vi "Loop_SM.vi"() -> ()   [LabVIEW 2017, in "MechamunDrive.lvlib"]
uses:
  MechamunDrive.lvlib
  Cluster_Auto Shut Off Ranges.ctl
  TypeDefs/Cluster_PID Constants Standard.ctl
  ENUM_State.ctl
  Enum_SM Cmd Select.ctl
  ENUM_Action.ctl
  Enum Tab_Select PID Mode.ctl
  Cluster_SM to HW Data.ctl
  Enum_HW Cmd Select.ctl
  Cluster_CMD to SM Data.ctl
  Cluster_HW Status.ctl
  TypeDefs/Cluster_SRX Status With Encoder.ctl
  VisionSystem/Cluster_Vision Status.ctl
  VisionSystem/Enum_ Field Targets.ctl
  Cluster_SM Status.ctl
  <vilib>/Rock Robotics/WPI/ThirdParty/Sensors/navX/_TypeDefs/FRIC_navX_DeviceNumbersTypeDef.ctl
  Global_CMD to SM Data.vi
  Sonar/Global_HW_Data Out.vi
  Global_HW_Status Out.vi
  VisionSystem/Global_Vision Status.vi
  _SHARE ALL/Global Share All/Global_STOP.vi
  <vilib>/addons/control/pid/pid.llb/PID (DBL).vi
  Global_SM Out Data.vi
  <vilib>/addons/control/pid/NI_PID_pid.lvlib
  Sonar/Sonar.lvlib
  VisionSystem/VisionSystem.lvlib
panel:
  out "Drive_HW_Status":T1
  out "SM Cmd":T3
  out "HW Cmd Out":T5
  in  "PID Select":T7
  in  "PID Track Rotation":T8={"proportional gain (Kc)"=0.005, "integral time (Ti, min)"=0.0, "derivative time (Td, min)"=0.0028} {"derivative time (Td, min)" format="%.5f"; "integral time (Ti, min)" format="%.5f"; "proportional gain (Kc)" format="%.5f"}
  in  "PID Lock Angle Rotation":T8={"proportional gain (Kc)"=0.012, "integral time (Ti, min)"=0.0, "derivative time (Td, min)"=0.002} {"derivative time (Td, min)" format="%.5f"; "integral time (Ti, min)" format="%.5f"; "proportional gain (Kc)" format="%.5f"}
  in  "PID Track Lateral":T8={"proportional gain (Kc)"=0.05, "integral time (Ti, min)"=0.0, "derivative time (Td, min)"=0.0} {"derivative time (Td, min)" format="%.5f"; "integral time (Ti, min)" format="%.5f"; "proportional gain (Kc)" format="%.5f"}
  in  "PID Track Vision Lat":T8={"proportional gain (Kc)"=0.03, "integral time (Ti, min)"=0.0, "derivative time (Td, min)"=0.0} {"derivative time (Td, min)" format="%.5f"; "integral time (Ti, min)" format="%.5f"; "proportional gain (Kc)" format="%.5f"}
  in  "lateral f":dbl=0.1 format="%#_13g"
  in  "PID Track Vision Rot":T8={"proportional gain (Kc)"=0.0015, "integral time (Ti, min)"=0.0, "derivative time (Td, min)"=0.0} {"derivative time (Td, min)" format="%.5f"; "integral time (Ti, min)" format="%.5f"; "proportional gain (Kc)" format="%.5f"}
  in  "Vision Track target":dbl=8.0 format="%#_13g"
  in  "PID Track Front":T8={"proportional gain (Kc)"=0.005, "integral time (Ti, min)"=0.0, "derivative time (Td, min)"=0.0} {"derivative time (Td, min)" format="%.5f"; "integral time (Ti, min)" format="%.5f"; "proportional gain (Kc)" format="%.5f"}
  out "Action":T9
  out "CMDMODE":T4
  out "Complete":bool
  out "PID Output":dbl
  out "PID Reading":dbl
  out "PID Target":dbl
  out "Cycle Time":dbl
  out "State":T10
  out "Output":dbl(graph)
  out "Process Chart":cluster{"PID Target":dbl, "PID Reading":dbl}(graph)
  in  "Auto Shut Off Ranges":T11={"Track Front Back"=1.0, "Track Rotation"=1.0, "Track Lateral"=1.0, "Track Vision"=2.0}
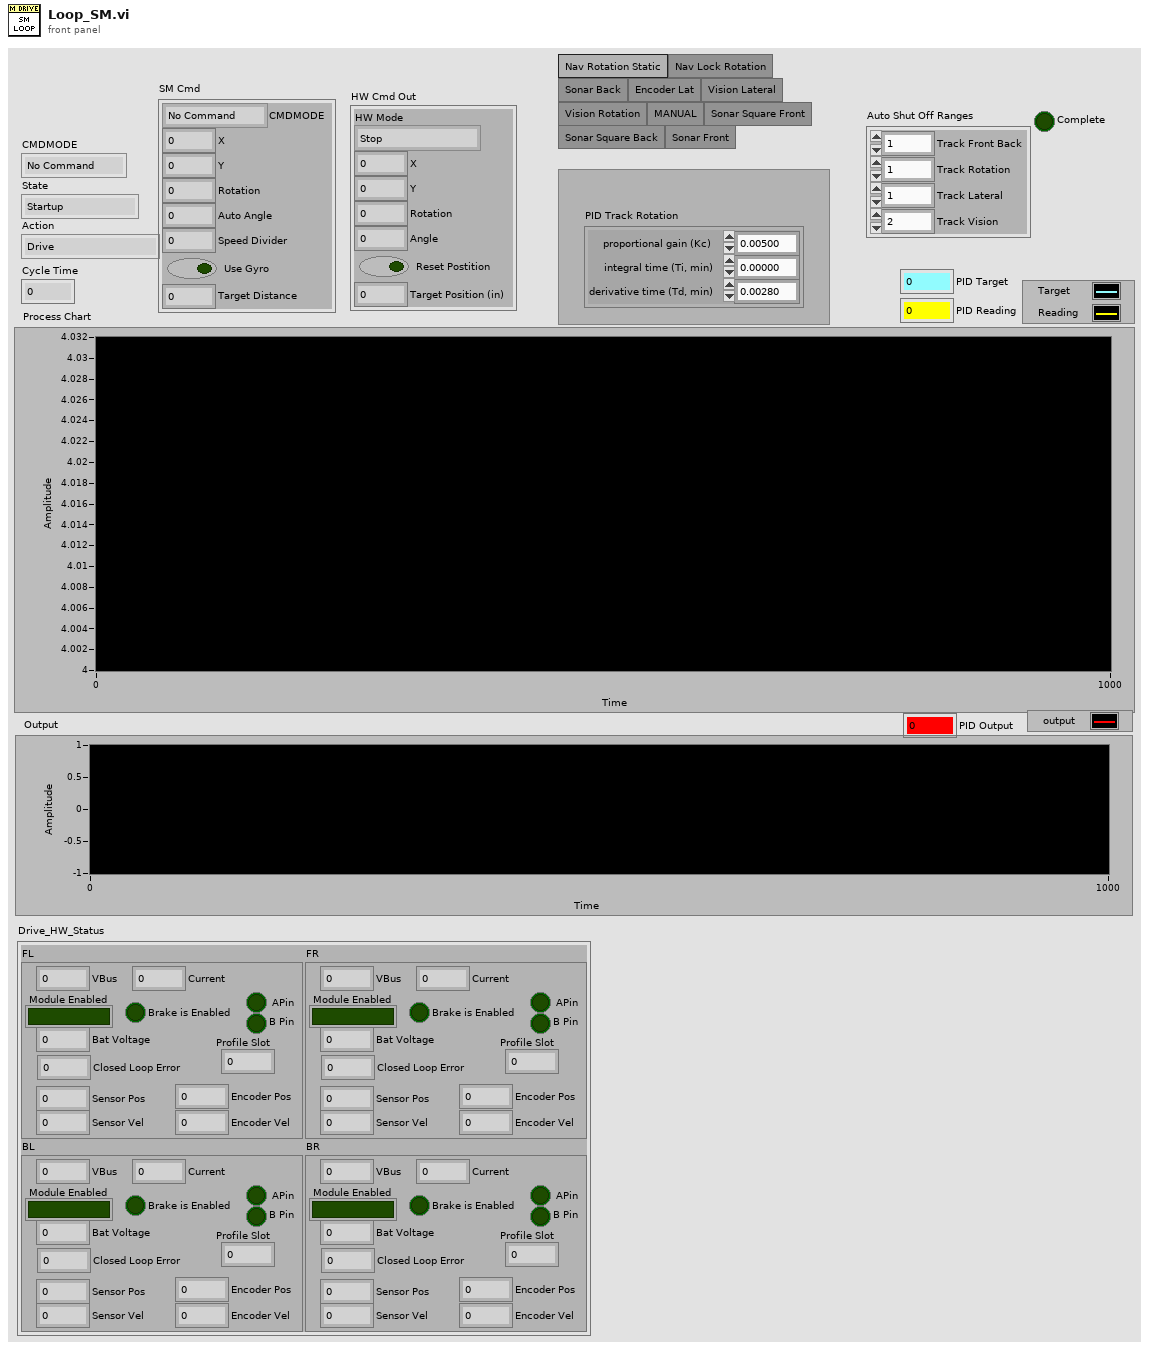
[diagram p1: front panel]
types:
  T1 = typedef "MechamunDrive.lvlib/Cluster_HW Status.ctl" = cluster{"BL":T2, "BR":T2, "FL":T2, "FR":T2}
  T2 = typedef "Cluster_SRX Status With Encoder.ctl" = cluster{"VBus ":dbl, "Module Enabled":bool, "Closed Loop Error":dbl, "Sensor Pos":dbl, "Sensor Vel":dbl, "Current":dbl, "Brake is Enabled":bool, "Encoder Pos":dbl, "Encoder Vel":dbl, " APin":bool, "B Pin":bool, "Bat Voltage":dbl, "Profile Slot":dbl}
  T3 = typedef "MechamunDrive.lvlib/Cluster_CMD to SM Data.ctl" = cluster{"CMDMODE":T4, "X":dbl, "Y":dbl, "Rotation":dbl, "Auto Angle":dbl, "Speed Divider":dbl, "Use Gyro":bool, "Target Distance":dbl}
  T4 = typedef "MechamunDrive.lvlib/Enum_SM Cmd Select.ctl" = enum16{"No Command", "Halt", "Manual Keep Rotation", "Manual", "Track Front", "Track Rotation", "Track Lateral", "Track Vision Lat", "Track Vision Rot", "Strafe Right", "Strafe Left"}
  T5 = typedef "MechamunDrive.lvlib/Cluster_SM to HW Data.ctl" = cluster{"HW Mode":T6, "X":dbl, "Y":dbl, "Rotation":dbl, "Angle":dbl, "Reset Postition":bool, "Target Position (in)":dbl}
  T6 = typedef "MechamunDrive.lvlib/Enum_HW Cmd Select.ctl" = enum16{"Stop", "Vbus", "Positon Lateral", "Postition  FrontBack"}
  T7 = typedef "MechamunDrive.lvlib/Enum Tab_Select PID Mode.ctl" = enum32{"Nav Rotation Static", "Nav Lock Rotation", "Sonar Back", "Encoder Lat", "Vision Lateral", "Vision Rotation", "MANUAL", "Sonar Square Front", "Sonar Square Back", "Sonar Front"}
  T8 = typedef "Cluster_PID Constants Standard.ctl" = cluster{"proportional gain (Kc)":dbl, "integral time (Ti, min)":dbl, "derivative time (Td, min)":dbl}
  T9 = typedef "MechamunDrive.lvlib/ENUM_Action.ctl" = enum16{"Drive", "Strafe Left", "Strafe Right", "No Action", "Manuel Keep Rotation", "Reset Time", "Stop Move", "Track Front Distance", "Set Lock Angle", "Reset Gyro", "Track Rotation", "Track Lateral Encoders", "NavX Pos Reset", "Track Vision Lat", "Track Vision Rot", "Reset Position"}
  T10 = typedef "MechamunDrive.lvlib/ENUM_State.ctl" = enum16{"Startup", "Idle", "Manual", "Rotation Tracking", "Distance Tracking", "Shutdown", "Lateral Tracking", "Vision Tracking Lat", "Vision Tracking Rot", "Strafing", "Manual Keep Rotation", "Halt"}
  T11 = typedef "MechamunDrive.lvlib/Cluster_Auto Shut Off Ranges.ctl" = cluster{"Track Front Back":dbl, "Track Rotation":dbl, "Track Lateral":dbl, "Track Vision":dbl}
  T12 = typedef "MechamunDrive.lvlib/Cluster_SM Status.ctl" = cluster{"Drive Cmd":T4, "Complete":bool}
  T13 = typedef "VisionSystem.lvlib/Cluster_Vision Status.ctl" = cluster{"Target Found":bool, "Target":T14, "Pixels to Center":dbl, "Vision Distance Center (in)":dbl, "Angle Distance Center (in)":dbl}
  T14 = typedef "VisionSystem.lvlib/Enum_ Field Targets.ctl" = enum16{"Boiler (USB 0)", "Rope (USB 1)"}
  T15 = cluster{"Velocity X":dbl, "Velocity Y":dbl, "Velocity Z":dbl, "Displacement X":dbl, "Displacement Y":dbl, "Displacement Z":dbl}
  T16 = cluster{"Actions":T9[], "State":T10, "Current Time":timestamp, "Start Time":timestamp, "Loop Time (ms)":u32, "CMD Drive":T3, "Set Angle Out":dbl, "Sonar Distance":dbl, "Lock Angle":dbl, "previous State":T10, "Position Data":cluster{"Velocity X":dbl, "Velocity Y":dbl, "Velocity Z":dbl, "Displacement X":dbl, "Displacement Y":dbl, "Displacement Z":dbl}, "Vision Data":T13, "Shut Off Ranges":T11, "Status OUT":T12, "PID Target":dbl, "PID Reading":dbl, "PID Output":dbl, "DriveHWCmd OUT":T5, "Gyro Angle":dbl, "Drive HW Status":T1, "Lateral Distance":dbl, "PID Select":T7}
  T17 = typedef "FRIC_navX_DeviceNumbersTypeDef.ctl" = enum16{"Dev0", "Dev1", "Dev2", "Dev3"}
  T18 = cluster{"Yaw":dbl, "Roll":dbl, "Pitch":dbl, "Heading":dbl, "Fused Heading":dbl}
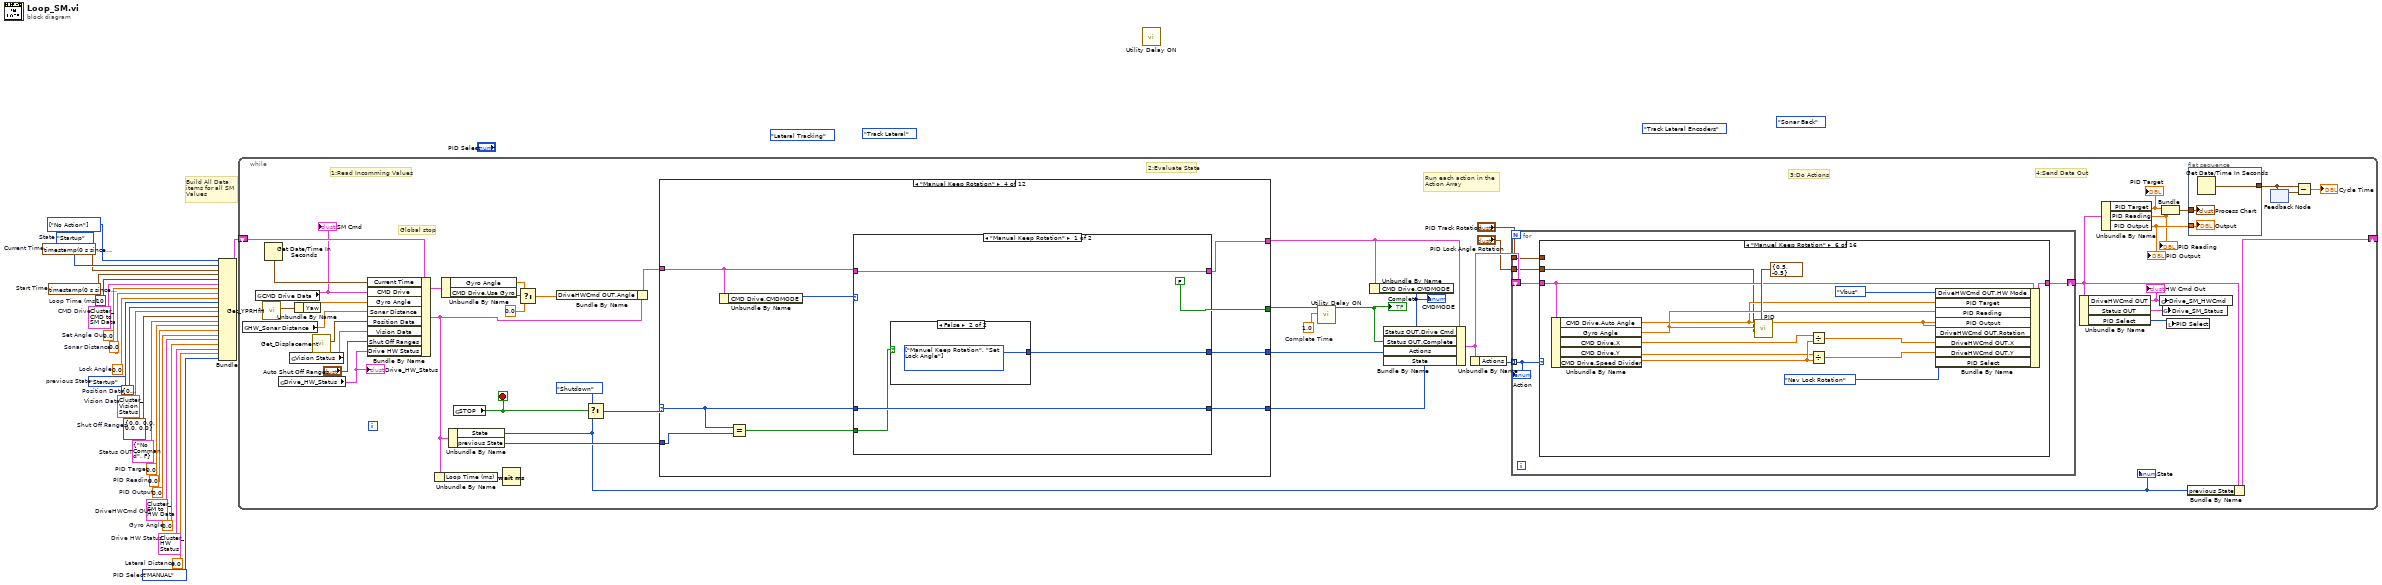
[diagram p0: block diagram]
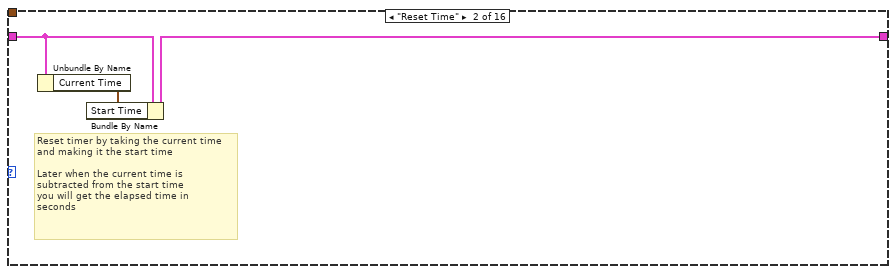
[diagram p3: hidden frame]
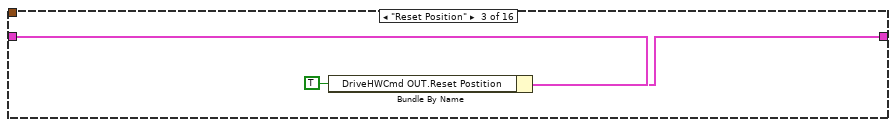
[diagram p4: hidden frame]
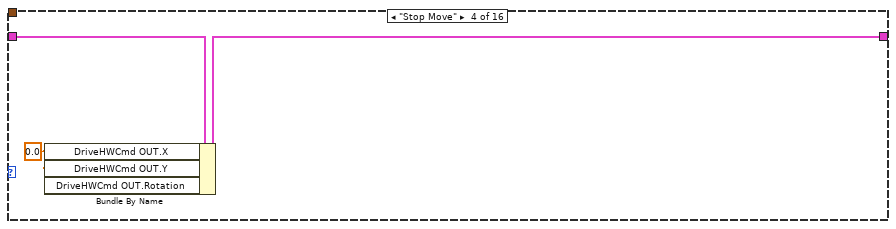
[diagram p5: hidden frame]
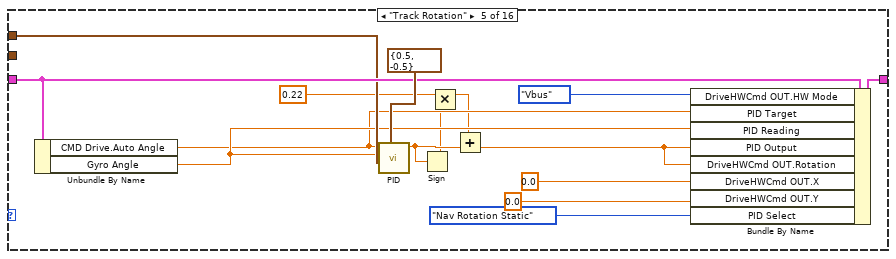
[diagram p6: hidden frame]
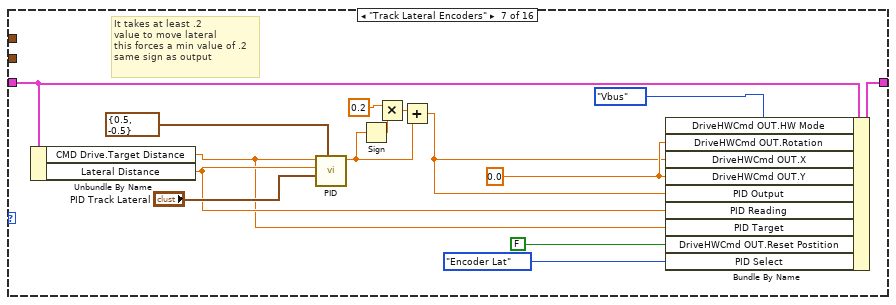
[diagram p7: hidden frame]
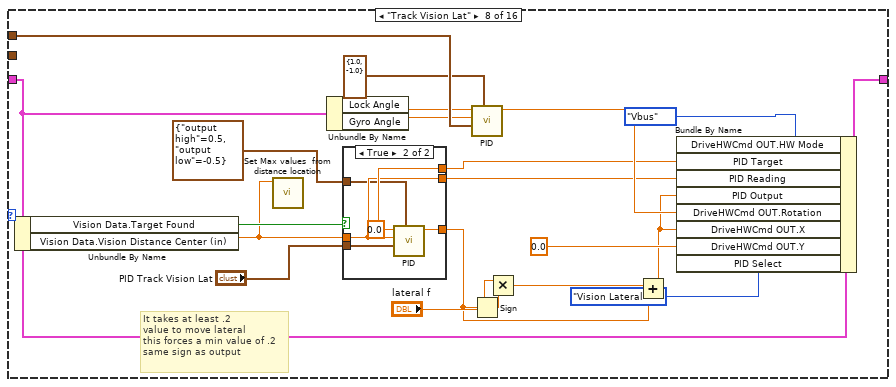
[diagram p8: hidden frame]
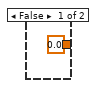
[diagram p9: hidden frame]
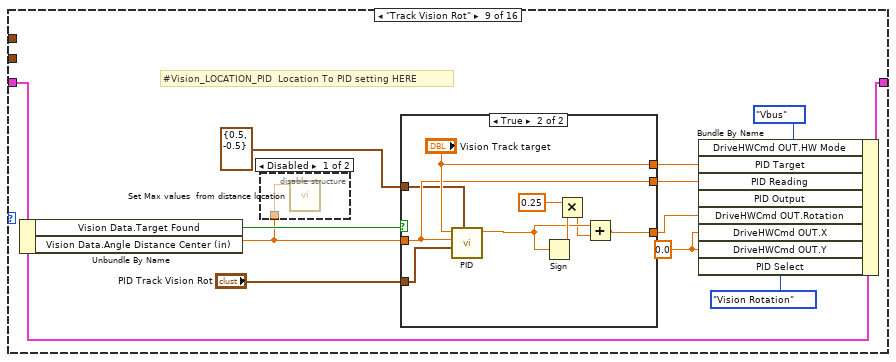
[diagram p10: hidden frame]
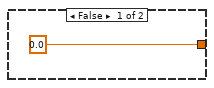
[diagram p12: hidden frame]
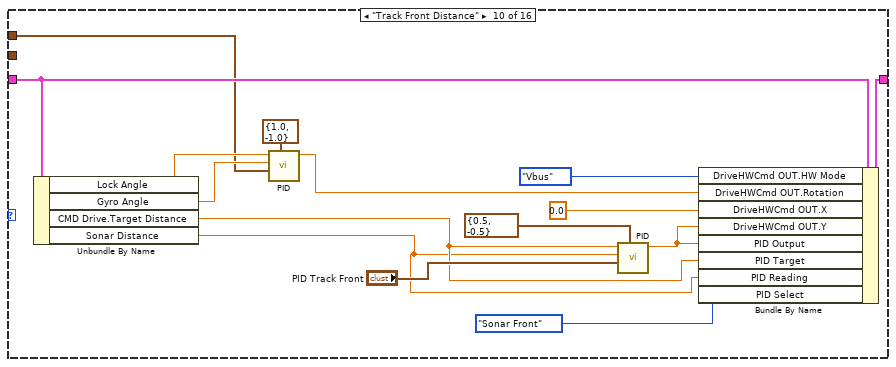
[diagram p13: hidden frame]
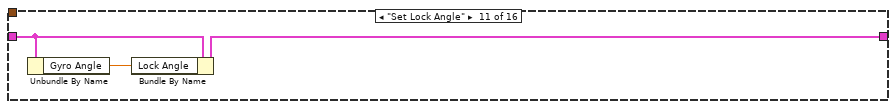
[diagram p14: hidden frame]
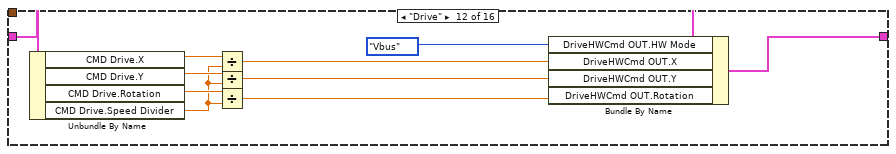
[diagram p15: hidden frame]
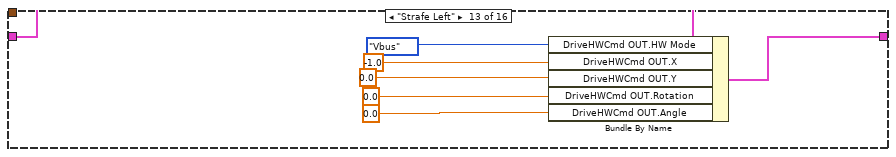
[diagram p16: hidden frame]
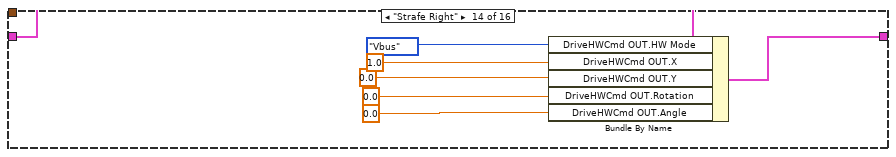
[diagram p17: hidden frame]
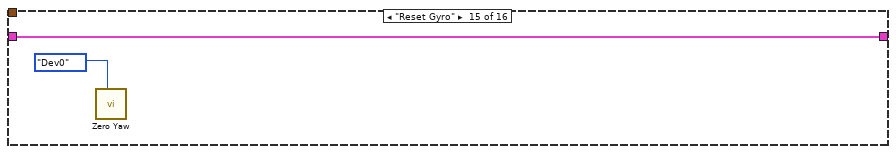
[diagram p18: hidden frame]
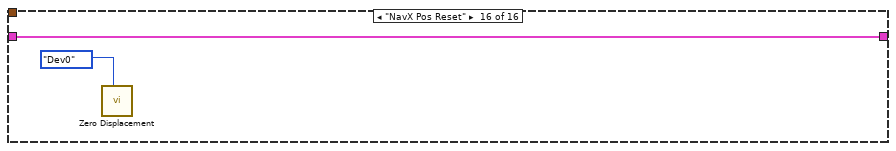
[diagram p19: hidden frame]
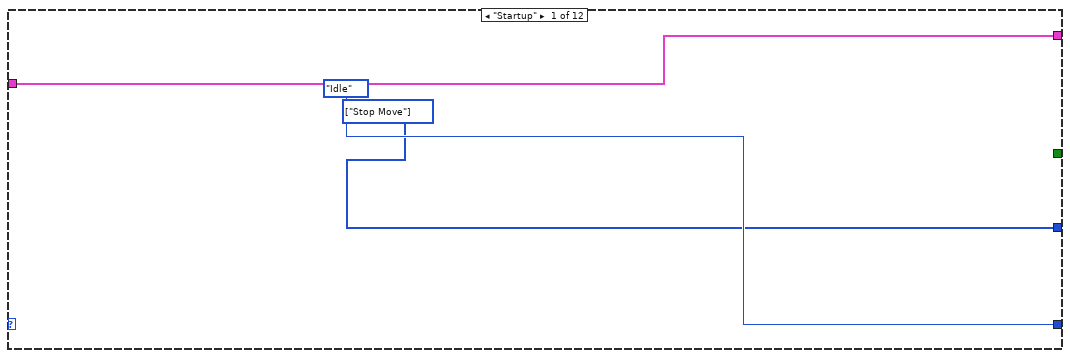
[diagram p20: hidden frame]
diagram:
  (unwired) Enum_SM_Cmd_Select."Track Lateral" ("CMD Drive.CMDMODE")
  (unwired) Enum_Tab_Select_PID_Mode."Sonar Back" ("PID Select")
  (unwired) ENUM_Action."Track Lateral Encoders" ("Action")
  (unwired) ENUM_State."Lateral Tracking" ("State")
  w1 = 0.0  # Sonar Distance
  w2 = Enum_Tab_Select_PID_Mode."MANUAL"  # PID Select
  w3 = 0.0  # Lateral Distance
  w4 = T1 {"BL"={"VBus "=0.0, "Module Enabled"=FALSE, "Closed Loop Error"=0.0, "Sensor Pos"=0.0, "Sensor Vel"=0.0, "Current"=0.0, "Brake is Enabled"=FALSE, "Encoder Pos"=0.0, "Encoder Vel"=0.0, " APin"=FALSE, "B Pin"=FALSE, "Bat Voltage"=0.0, "Profile Slot"=0.0}, "BR"={"VBus "=0.0, "Module Enabled"=FALSE, "Closed Loop Error"=0.0, "Sensor Pos"=0.0, "Sensor Vel"=0.0, "Current"=0.0, "Brake is Enabled"=FALSE, "Encoder Pos"=0.0, "Encoder Vel"=0.0, " APin"=FALSE, "B Pin"=FALSE, "Bat Voltage"=0.0, "Profile Slot"=0.0}, "FL"={"VBus "=0.0, "Module Enabled"=FALSE, "Closed Loop Error"=0.0, "Sensor Pos"=0.0, "Sensor Vel"=0.0, "Current"=0.0, "Brake is Enabled"=FALSE, "Encoder Pos"=0.0, "Encoder Vel"=0.0, " APin"=FALSE, "B Pin"=FALSE, "Bat Voltage"=0.0, "Profile Slot"=0.0}, "FR"={"VBus "=0.0, "Module Enabled"=FALSE, "Closed Loop Error"=0.0, "Sensor Pos"=0.0, "Sensor Vel"=0.0, "Current"=0.0, "Brake is Enabled"=FALSE, "Encoder Pos"=0.0, "Encoder Vel"=0.0, " APin"=FALSE, "B Pin"=FALSE, "Bat Voltage"=0.0, "Profile Slot"=0.0}}  # Drive HW Status
  w5 = 0.0  # Gyro Angle
  w6 = T5 {"HW Mode"=enum."Postition  FrontBack", "X"=0.0, "Y"=0.0, "Rotation"=0.0, "Angle"=0.0, "Reset Postition"=FALSE, "Target Position (in)"=0.0}  # DriveHWCmd OUT
  w7 = 0.0  # PID Output
  w8 = 0.0  # PID Reading
  w9 = 0.0  # PID Target
  w10 = T12 {"Drive Cmd"=enum."No Command", "Complete"=FALSE}  # Status OUT
  w11 = T11 {"Track Front Back"=0.0, "Track Rotation"=0.0, "Track Lateral"=0.0, "Track Vision"=0.0}  # Shut Off Ranges
  w12 = T13 {"Target Found"=FALSE, "Target"=enum."Boiler (USB 0)", "Pixels to Center"=0.0, "Vision Distance Center (in)"=0.0, "Angle Distance Center (in)"=0.0}  # Vision Data
  w13 = T15 {"Velocity X"=0.0, "Velocity Y"=0.0, "Velocity Z"=0.0, "Displacement X"=0.0, "Displacement Y"=0.0, "Displacement Z"=0.0}  # Position Data
  w14 = ENUM_State."Startup"  # previous State
  w15 = 0.0  # Lock Angle
  w16 = 0.0  # Set Angle Out
  w17 = T3 {"CMDMODE"=enum."No Command", "X"=0.0, "Y"=0.0, "Rotation"=0.0, "Auto Angle"=0.0, "Speed Divider"=0.0, "Use Gyro"=FALSE, "Target Distance"=0.0}  # CMD Drive
  w18 = u32 10  # Loop Time (ms)
  w19 = T9[] [enum."No Action"] items=["Drive", "Strafe Left", "Strafe Right", "No Action", "Manuel Keep Rotation", "Reset Time", "Stop Move", "Track Front Distance", "Set Lock Angle", "Reset Gyro", "Track Rotation", "Track Lateral Encoders", "NavX Pos Reset", "Track Vision Lat", "Track Vision Rot", "Reset Position"] ("Actions")
  w20 = timestamp(0 s since 1904-01-01)  # Start Time
  w21 = timestamp(0 s since 1904-01-01)  # Current Time
  w22 = ENUM_State."Startup"  # State
  # "Build All Data items for all SM Values"
  n1 = Bundle("Actions"=w19, "State"=w22, "Current Time"=w21, "Start Time"=w20, "Loop Time (ms)"=w18, "CMD Drive"=w17, "Set Angle Out"=w16, "Sonar Distance"=w1, "Lock Angle"=w15, "previous State"=w14, "Position Data"=w13, "Vision Data"=w12, "Shut Off Ranges"=w11, "Status OUT"=w10, "PID Target"=w9, "PID Reading"=w8, "PID Output"=w7, "DriveHWCmd OUT"=w6, "Gyro Angle"=w5, "Drive HW Status"=w4, "Lateral Distance"=w3, "PID Select"=w2) -> (w23:T16)  [unwired: 1 in]
  n2 = while {
    shift-right: [w48] -> _
    shift-left: w23 -> [w67]
    stop <- w64 stop-if-true
    w24 = 1.0  # Complete Time
    # "Run each action in the Action Array"
    # "1:Read Incomming Values"
    # "2:Evaluate State"
    # "3:Do Actions"
    # "4:Send Data Out"
    # "Global stop"
    n3 = global read "Global_HW_Data Out.vi" "HW_Sonar Distance"() -> (w27:dbl)
    n4 = global read "Global_CMD to SM Data.vi" "CMD Drive Data"() -> (w60:T3)
    "SM Cmd" <- w60
    n5 = call <vilib>:"Get_YPRHfH.vi"() -> ("YRPHfH"=w59:T18)  [unwired: 11 in]
    n6 = Get Date/Time In Seconds() -> (seconds since 1Jan1904=w66:timestamp)
    n7 = global read "Global_HW_Status Out.vi" "Drive_HW_Status"() -> (w29:T1)
    "Drive_HW_Status" <- w29
    n8 = global read "Global_Vision Status.vi" "Vision Status"() -> (w46:T13)
    n9 = Unbundle By Name(w59) -> ("Yaw"=w57:dbl)
    n10 = call <vilib>:"Get_Displacement.vi"() -> ("Displacement"=w47:T15)  [unwired: 11 in]
    n11 = Bundle By Name(cluster=w67, "Current Time"=w66, "CMD Drive"=w60, "Gyro Angle"=w57, "Sonar Distance"=w27, "Position Data"=w47, "Vision Data"=w46, "Shut Off Ranges"="Auto Shut Off Ranges", "Drive HW Status"=w29) -> (w52:T16)
    n12 = Unbundle By Name(w52) -> ("Loop Time (ms)"=w61:u32)
    n13 = Unbundle By Name(w52) -> ("Gyro Angle"=w54:dbl, "CMD Drive.Use Gyro"=w55:bool)
    n14 = Unbundle By Name(w52) -> ("State"=w45:T10, "previous State"=w49:T10)
    "State" <- w45
    n15 = global read "Global_STOP.vi" "STOP"() -> (w64:bool)
    n16 = Wait (ms)(milliseconds to wait=w61) -> ()  [unwired: 1 out]
    n17 = Select(t=w54, s=w55, f=0.0) -> (s? t:f=w50:dbl)
    n18 = Bundle By Name(cluster=w52, "DriveHWCmd OUT.Angle"=w50) -> (w51:T16)
    n19 = Select(t=ENUM_State."Shutdown" ("State"), s=w64, f=w45) -> (s? t:f=w62:T10)
    n20 = case shown="\"Manual Keep Rotation\"" w62 {
      selector: w62 -> [_ _ w260 w271 w287 w309 w352 w386 w412 _ _ _]
      tunnel: w51 -> [w229 w232 w256 w272 w292 w314 w357 w391 w416 w434 w438 w446]
      tunnel: [w229 w231 w257 w273 w291 w315 w358 w392 w415 w434 w438 w446] -> w42
      tunnel: [ENUM_State."Idle" ("State") w230 w259 w275 w290 w313 w356 w390 w411 ENUM_State."Shutdown" ("State") w435 w445] -> w40
      tunnel: [w227 _ w258 w274 w289 w312 w355 w389 w413 w432 w436 w448] -> w58
      tunnel: w49 -> [_ _ _ w270 _ w310 w353 w387 _ _ _ _]
      tunnel: [_ _ FALSE FALSE w288 w311 w354 w388 w414 _ _ _] -> w25
      frame "Startup" {
        w227 = T9[] [enum."Stop Move"] items=["Drive", "Strafe Left", "Strafe Right", "No Action", "Manuel Keep Rotation", "Reset Time", "Stop Move", "Track Front Distance", "Set Lock Angle", "Reset Gyro", "Track Rotation", "Track Lateral Encoders", "NavX Pos Reset", "Track Vision Lat", "Track Vision Rot", "Reset Position"] ("Actions")
      }
      frame "Idle" {
        # "For each call of the state\nDecide next State and set\nActions"
        # "What will the next state be"
        n21 = Unbundle By Name(w232) -> ("CMD Drive.CMDMODE"=w233:T4)
        n22 = case shown="\"Halt\"" w233 {
          tunnel: w232 -> [w234 w236 w239 w240 w243 w245 w247 w249 w250 w253 w255]
          tunnel: [w234 w236 w239 w240 w243 w245 w247 w249 w250 w253 w255] -> w231
          tunnel: [ENUM_State."Idle" ("State") ENUM_State."Rotation Tracking" ("State") ENUM_State."Manual Keep Rotation" ("State") ENUM_State."Distance Tracking" ("State") ENUM_State."Lateral Tracking" ("State") ENUM_State."Manual" ("State") ENUM_State."Vision Tracking Lat" ("State") ENUM_State."Vision Tracking Rot" ("State") ENUM_State."Strafing" ("State") ENUM_State."Strafing" ("State") ENUM_State."Halt" ("State")] -> w230
          frame "No Command" {
          }
          frame "Track Rotation" {
          }
          frame "Manual Keep Rotation" {
          }
          frame "Track Front" {
          }
          frame "Track Lateral" {
          }
          frame "Manual" {
          }
          frame "Track Vision Lat" {
          }
          frame "Track Vision Rot" {
          }
          frame "Strafe Right" {
          }
          frame "Strafe Left" {
          }
          frame "Halt" {
          }
        }
      }
      frame "Manual" {
        n23 = Unbundle By Name(w256) -> ("CMD Drive.CMDMODE"=w261:T4)
        n24 = case shown="\"Manual\"" w261 {
          tunnel: w256 -> [w264 w268]
          tunnel: [w264 w268] -> w257
          tunnel: [w263 ENUM_State."Idle" ("State")] -> w259
          tunnel: [w265 w266] -> w258
          tunnel: w260 -> [w263 _]
          frame "Manual" {
            w265 = T9[] [enum."Drive"] items=["Drive", "Strafe Left", "Strafe Right", "No Action", "Manuel Keep Rotation", "Reset Time", "Stop Move", "Track Front Distance", "Set Lock Angle", "Reset Gyro", "Track Rotation", "Track Lateral Encoders", "NavX Pos Reset", "Track Vision Lat", "Track Vision Rot", "Reset Position"] ("Actions")
          }
          frame Default {
            w266 = T9[] [enum."Stop Move"] items=["Drive", "Strafe Left", "Strafe Right", "No Action", "Manuel Keep Rotation", "Reset Time", "Stop Move", "Track Front Distance", "Set Lock Angle", "Reset Gyro", "Track Rotation", "Track Lateral Encoders", "NavX Pos Reset", "Track Vision Lat", "Track Vision Rot", "Reset Position"] ("Actions")
          }
        }
      }
      frame "Manual Keep Rotation" {
        n25 = Unbundle By Name(w272) -> ("CMD Drive.CMDMODE"=w276:T4)
        n26 = Equal?(x=w271, y=w270) -> (x = y?=w269:bool)
        n27 = case shown="\"Manual Keep Rotation\"" w276 {
          tunnel: w272 -> [w280 w286]
          tunnel: [w280 w286] -> w273
          tunnel: [w279 ENUM_State."Idle" ("State")] -> w275
          tunnel: [w281 w284] -> w274
          tunnel: w271 -> [w279 _]
          tunnel: w269 -> [w278 _]
          frame "Manual Keep Rotation" {
            n28 = case shown="False" w278 {
              tunnel: [w282 w283] -> w281
              frame True {
                w282 = T9[] [enum."Manuel Keep Rotation"] items=["Drive", "Strafe Left", "Strafe Right", "No Action", "Manuel Keep Rotation", "Reset Time", "Stop Move", "Track Front Distance", "Set Lock Angle", "Reset Gyro", "Track Rotation", "Track Lateral Encoders", "NavX Pos Reset", "Track Vision Lat", "Track Vision Rot", "Reset Position"] ("Actions")
              }
              frame False {
                w283 = T9[] [enum."Manuel Keep Rotation", enum."Set Lock Angle"] items=["Drive", "Strafe Left", "Strafe Right", "No Action", "Manuel Keep Rotation", "Reset Time", "Stop Move", "Track Front Distance", "Set Lock Angle", "Reset Gyro", "Track Rotation", "Track Lateral Encoders", "NavX Pos Reset", "Track Vision Lat", "Track Vision Rot", "Reset Position"] ("Actions")
              }
            }
          }
          frame Default {
            w284 = T9[] [enum."Stop Move"] items=["Drive", "Strafe Left", "Strafe Right", "No Action", "Manuel Keep Rotation", "Reset Time", "Stop Move", "Track Front Distance", "Set Lock Angle", "Reset Gyro", "Track Rotation", "Track Lateral Encoders", "NavX Pos Reset", "Track Vision Lat", "Track Vision Rot", "Reset Position"] ("Actions")
          }
        }
      }
      frame "Rotation Tracking" {
        n29 = Unbundle By Name(w292) -> ("CMD Drive.CMDMODE"=w293:T4)
        n30 = case shown="Default" w293 {
          tunnel: w292 -> [w295 w307]
          tunnel: [w295 w307] -> w291
          tunnel: [w297 ENUM_State."Idle" ("State")] -> w290
          tunnel: [w296 w305] -> w289
          tunnel: [w294 _] -> w288
          tunnel: w287 -> [w297 _]
          frame "Track Rotation" {
            n31 = Unbundle By Name(w295) -> ("CMD Drive.Auto Angle"=w301:dbl, "Gyro Angle"=w302:dbl, "Shut Off Ranges.Track Rotation"=w299:dbl)
            n32 = Subtract(x=w301, y=w302) -> (x-y=w300:dbl)
            n33 = Absolute Value(x=w300) -> (abs(x)=w298:dbl)
            n34 = Less Or Equal?(x=w298, y=w299) -> (x <= y?=w294:bool)
            n35 = case shown="True" w294 {
              tunnel: [w303 w304] -> w296
              frame False {
                w303 = T9[] [enum."Track Rotation"] items=["Drive", "Strafe Left", "Strafe Right", "No Action", "Manuel Keep Rotation", "Reset Time", "Stop Move", "Track Front Distance", "Set Lock Angle", "Reset Gyro", "Track Rotation", "Track Lateral Encoders", "NavX Pos Reset", "Track Vision Lat", "Track Vision Rot", "Reset Position"] ("Actions")
              }
              frame True {
                w304 = T9[] [enum."Stop Move"] items=["Drive", "Strafe Left", "Strafe Right", "No Action", "Manuel Keep Rotation", "Reset Time", "Stop Move", "Track Front Distance", "Set Lock Angle", "Reset Gyro", "Track Rotation", "Track Lateral Encoders", "NavX Pos Reset", "Track Vision Lat", "Track Vision Rot", "Reset Position"] ("Actions")
              }
            }
          }
          frame Default {
            w305 = T9[] [enum."Stop Move"] items=["Drive", "Strafe Left", "Strafe Right", "No Action", "Manuel Keep Rotation", "Reset Time", "Stop Move", "Track Front Distance", "Set Lock Angle", "Reset Gyro", "Track Rotation", "Track Lateral Encoders", "NavX Pos Reset", "Track Vision Lat", "Track Vision Rot", "Reset Position"] ("Actions")
          }
        }
      }
      frame "Lateral Tracking" {
        n36 = Unbundle By Name(w314) -> ("CMD Drive.CMDMODE"=w316:T4)
        n37 = Not Equal?(x=w309, y=w310) -> (x != y?=w308:bool)
        n38 = case shown="\"Track Lateral\"" w316 {
          tunnel: w314 -> [w319 w350]
          tunnel: [w318 w350] -> w315
          tunnel: [w321 ENUM_State."Idle" ("State")] -> w313
          tunnel: [w322 w348] -> w312
          tunnel: [w320 _] -> w311
          tunnel: w309 -> [w321 _]
          tunnel: w308 -> [w317 _]
          frame "Track Lateral" {
            n39 = case shown="False" w317 {
              tunnel: [w330 w347] -> w322
              tunnel: [w329 FALSE] -> w320
              tunnel: w319 -> [w325 w346]
              tunnel: [w327 w346] -> w318
              frame False {
                # "Previous \nSame"
                n40 = Unbundle By Name(w325) -> ("Drive HW Status"=w328:T1)
                n41 = call "Calculate Position.vi"("Drive HW Status"=w328) -> ("Reset"=w326:bool, "Distance"=w323:dbl)  [unwired: 8 in, 1 out]
                n42 = Bundle By Name(cluster=w325, "Lateral Distance"=w323) -> (w324:T16)
                n43 = case shown="False" w326 {
                  tunnel: [w339 w343] -> w330
                  tunnel: w324 -> [w332 w344]
                  tunnel: [w333 _] -> w329
                  tunnel: [w332 w344] -> w327
                  tunnel: w323 -> [w331 _]
                  frame False {
                    # "Encoders have value"
                    n44 = Unbundle By Name(w332) -> ("CMD Drive.Target Distance"=w338:dbl, "Shut Off Ranges.Track Lateral"=w336:dbl)
                    n45 = Subtract(x=w338, y=w331) -> (x-y=w337:dbl)
                    n46 = Absolute Value(x=w337) -> (abs(x)=w334:dbl)
                    n47 = Less Or Equal?(x=w334, y=w336) -> (x <= y?=w335:bool)
                    n48 = case shown="False" w335 {
                      tunnel: [w340 w342] -> w339
                      tunnel: [_ TRUE] -> w333
                      frame False {
                        w340 = T9[] [enum."Track Lateral Encoders"] items=["Drive", "Strafe Left", "Strafe Right", "No Action", "Manuel Keep Rotation", "Reset Time", "Stop Move", "Track Front Distance", "Set Lock Angle", "Reset Gyro", "Track Rotation", "Track Lateral Encoders", "NavX Pos Reset", "Track Vision Lat", "Track Vision Rot", "Reset Position"] ("Actions")
                      }
                      frame True {
                        w342 = T9[] [enum."Stop Move"] items=["Drive", "Strafe Left", "Strafe Right", "No Action", "Manuel Keep Rotation", "Reset Time", "Stop Move", "Track Front Distance", "Set Lock Angle", "Reset Gyro", "Track Rotation", "Track Lateral Encoders", "NavX Pos Reset", "Track Vision Lat", "Track Vision Rot", "Reset Position"] ("Actions")
                      }
                    }
                  }
                  frame True {
                    w343 = T9[] [enum."Drive", enum."Track Lateral Encoders"] items=["Drive", "Strafe Left", "Strafe Right", "No Action", "Manuel Keep Rotation", "Reset Time", "Stop Move", "Track Front Distance", "Set Lock Angle", "Reset Gyro", "Track Rotation", "Track Lateral Encoders", "NavX Pos Reset", "Track Vision Lat", "Track Vision Rot", "Reset Position"] ("Actions")
                    # "Encoder are Reset"
                  }
                }
              }
              frame True {
                w347 = T9[] [enum."Reset Position"] items=["Drive", "Strafe Left", "Strafe Right", "No Action", "Manuel Keep Rotation", "Reset Time", "Stop Move", "Track Front Distance", "Set Lock Angle", "Reset Gyro", "Track Rotation", "Track Lateral Encoders", "NavX Pos Reset", "Track Vision Lat", "Track Vision Rot", "Reset Position"] ("Actions")
                # "Initial Command"
              }
            }
          }
          frame Default {
            w348 = T9[] [enum."Stop Move"] items=["Drive", "Strafe Left", "Strafe Right", "No Action", "Manuel Keep Rotation", "Reset Time", "Stop Move", "Track Front Distance", "Set Lock Angle", "Reset Gyro", "Track Rotation", "Track Lateral Encoders", "NavX Pos Reset", "Track Vision Lat", "Track Vision Rot", "Reset Position"] ("Actions")
          }
        }
      }
      frame "Vision Tracking Lat" {
        n49 = Not Equal?(x=w352, y=w353) -> (x != y?=w351:bool)
        n50 = Unbundle By Name(w357) -> ("CMD Drive.CMDMODE"=w359:T4)
        n51 = case shown="\"Track Vision Lat\"" w359 {
          tunnel: w357 -> [w370 w384]
          tunnel: [w370 w384] -> w358
          tunnel: [w366 ENUM_State."Idle" ("State")] -> w356
          tunnel: [w371 w382] -> w355
          tunnel: [w364 _] -> w354
          tunnel: w352 -> [w366 _]
          tunnel: w351 -> [w365 _]
          frame "Track Vision Lat" {
            # "#VISION_ShutOFF_RANGES????"
            n52 = Unbundle By Name(w370) -> ("Vision Data.Target Found"=w361:bool, "Vision Data.Vision Distance Center (in)"=w363:dbl, "Shut Off Ranges.Track Vision"=w369:dbl)
            n53 = Absolute Value(x=w363) -> (abs(x)=w367:dbl)
            n54 = Not(x=w361) -> (.not. x?=w360:bool)
            n55 = Less Or Equal?(x=w367, y=w369) -> (x <= y?=w368:bool)
            n56 = Or(x=w360, y=w368) -> (x .or. y?=w362:bool)
            n57 = case shown="False" w362 {
              tunnel: [w373 w378] -> w371
              tunnel: w365 -> [w372 w377]
              tunnel: [_ w376] -> w364
              frame False {
                n58 = case shown="False" w372 {
                  tunnel: [w374 w375] -> w373
                  frame True {
                    w374 = T9[] [enum."NavX Pos Reset", enum."Set Lock Angle", enum."Track Vision Lat"] items=["Drive", "Strafe Left", "Strafe Right", "No Action", "Manuel Keep Rotation", "Reset Time", "Stop Move", "Track Front Distance", "Set Lock Angle", "Reset Gyro", "Track Rotation", "Track Lateral Encoders", "NavX Pos Reset", "Track Vision Lat", "Track Vision Rot", "Reset Position"] ("Actions")
                  }
                  frame False {
                    w375 = T9[] [enum."Track Vision Lat"] items=["Drive", "Strafe Left", "Strafe Right", "No Action", "Manuel Keep Rotation", "Reset Time", "Stop Move", "Track Front Distance", "Set Lock Angle", "Reset Gyro", "Track Rotation", "Track Lateral Encoders", "NavX Pos Reset", "Track Vision Lat", "Track Vision Rot", "Reset Position"] ("Actions")
                  }
                }
              }
              frame True {
                n59 = case shown="False" w377 {
                  tunnel: [w379 w381] -> w378
                  tunnel: [_ TRUE] -> w376
                  frame True {
                    w379 = T9[] [enum."NavX Pos Reset", enum."Set Lock Angle"] items=["Drive", "Strafe Left", "Strafe Right", "No Action", "Manuel Keep Rotation", "Reset Time", "Stop Move", "Track Front Distance", "Set Lock Angle", "Reset Gyro", "Track Rotation", "Track Lateral Encoders", "NavX Pos Reset", "Track Vision Lat", "Track Vision Rot", "Reset Position"] ("Actions")
                  }
                  frame False {
                    w381 = T9[] [enum."Stop Move"] items=["Drive", "Strafe Left", "Strafe Right", "No Action", "Manuel Keep Rotation", "Reset Time", "Stop Move", "Track Front Distance", "Set Lock Angle", "Reset Gyro", "Track Rotation", "Track Lateral Encoders", "NavX Pos Reset", "Track Vision Lat", "Track Vision Rot", "Reset Position"] ("Actions")
                  }
                }
              }
            }
          }
          frame Default {
            w382 = T9[] [enum."Stop Move"] items=["Drive", "Strafe Left", "Strafe Right", "No Action", "Manuel Keep Rotation", "Reset Time", "Stop Move", "Track Front Distance", "Set Lock Angle", "Reset Gyro", "Track Rotation", "Track Lateral Encoders", "NavX Pos Reset", "Track Vision Lat", "Track Vision Rot", "Reset Position"] ("Actions")
          }
        }
      }
      frame "Vision Tracking Rot" {
        n60 = Not Equal?(x=w386, y=w387) -> (x != y?=w385:bool)
        n61 = Unbundle By Name(w391) -> ("CMD Drive.CMDMODE"=w393:T4)
        n62 = case shown="\"Track Vision Rot\"" w393 {
          tunnel: w391 -> [w403 w410]
          tunnel: [w403 w410] -> w392
          tunnel: [w399 ENUM_State."Idle" ("State")] -> w390
          tunnel: [w404 w408] -> w389
          tunnel: [w398 _] -> w388
          tunnel: w386 -> [w399 _]
          tunnel: w385 -> [_ _]
          frame "Track Vision Rot" {
            n63 = Unbundle By Name(w403) -> ("Vision Data.Target Found"=w395:bool, "Vision Data.Angle Distance Center (in)"=w397:dbl, "Shut Off Ranges.Track Vision"=w402:dbl)
            n64 = Absolute Value(x=w397) -> (abs(x)=w400:dbl)
            n65 = Not(x=w395) -> (.not. x?=w394:bool)
            n66 = Less Or Equal?(x=w400, y=w402) -> (x <= y?=w401:bool)
            n67 = Or(x=w394, y=w401) -> (x .or. y?=w396:bool)
            n68 = case shown="True" w396 {
              tunnel: [w405 w407] -> w404
              tunnel: [_ TRUE] -> w398
              frame False {
                w405 = T9[] [enum."Track Vision Rot"] items=["Drive", "Strafe Left", "Strafe Right", "No Action", "Manuel Keep Rotation", "Reset Time", "Stop Move", "Track Front Distance", "Set Lock Angle", "Reset Gyro", "Track Rotation", "Track Lateral Encoders", "NavX Pos Reset", "Track Vision Lat", "Track Vision Rot", "Reset Position"] ("Actions")
              }
              frame True {
                w407 = T9[] [enum."Stop Move"] items=["Drive", "Strafe Left", "Strafe Right", "No Action", "Manuel Keep Rotation", "Reset Time", "Stop Move", "Track Front Distance", "Set Lock Angle", "Reset Gyro", "Track Rotation", "Track Lateral Encoders", "NavX Pos Reset", "Track Vision Lat", "Track Vision Rot", "Reset Position"] ("Actions")
              }
            }
          }
          frame Default {
            w408 = T9[] [enum."Stop Move"] items=["Drive", "Strafe Left", "Strafe Right", "No Action", "Manuel Keep Rotation", "Reset Time", "Stop Move", "Track Front Distance", "Set Lock Angle", "Reset Gyro", "Track Rotation", "Track Lateral Encoders", "NavX Pos Reset", "Track Vision Lat", "Track Vision Rot", "Reset Position"] ("Actions")
          }
        }
      }
      frame "Distance Tracking" {
        n69 = Unbundle By Name(w416) -> ("CMD Drive.CMDMODE"=w417:T4)
        n70 = case shown="\"Track Front\"" w417 {
          tunnel: w416 -> [w425 w431]
          tunnel: [w425 w431] -> w415
          tunnel: [w420 ENUM_State."Idle" ("State")] -> w411
          tunnel: [w426 w429] -> w413
          tunnel: [w422 _] -> w414
          tunnel: w412 -> [w420 _]
          frame "Track Front" {
            n71 = Unbundle By Name(w425) -> ("CMD Drive.Target Distance"=w424:dbl, "Sonar Distance"=w419:dbl, "Shut Off Ranges.Track Rotation"=w418:dbl)
            n72 = Subtract(x=w424, y=w419) -> (x-y=w423:dbl)
            n73 = Absolute Value(x=w423) -> (abs(x)=w421:dbl)
            n74 = Less Or Equal?(x=w421, y=w418) -> (x <= y?=w422:bool)
            n75 = case shown="False" w422 {
              tunnel: [w427 w428] -> w426
              frame False {
                w427 = T9[] [enum."Track Front Distance"] items=["Drive", "Strafe Left", "Strafe Right", "No Action", "Manuel Keep Rotation", "Reset Time", "Stop Move", "Track Front Distance", "Set Lock Angle", "Reset Gyro", "Track Rotation", "Track Lateral Encoders", "NavX Pos Reset", "Track Vision Lat", "Track Vision Rot", "Reset Position"] ("Actions")
              }
              frame True {
                w428 = T9[] [enum."Stop Move"] items=["Drive", "Strafe Left", "Strafe Right", "No Action", "Manuel Keep Rotation", "Reset Time", "Stop Move", "Track Front Distance", "Set Lock Angle", "Reset Gyro", "Track Rotation", "Track Lateral Encoders", "NavX Pos Reset", "Track Vision Lat", "Track Vision Rot", "Reset Position"] ("Actions")
              }
            }
          }
          frame Default {
            w429 = T9[] [enum."Stop Move"] items=["Drive", "Strafe Left", "Strafe Right", "No Action", "Manuel Keep Rotation", "Reset Time", "Stop Move", "Track Front Distance", "Set Lock Angle", "Reset Gyro", "Track Rotation", "Track Lateral Encoders", "NavX Pos Reset", "Track Vision Lat", "Track Vision Rot", "Reset Position"] ("Actions")
          }
        }
      }
      frame "Shutdown" {
        w432 = T9[] [enum."Stop Move"] items=["Drive", "Strafe Left", "Strafe Right", "No Action", "Manuel Keep Rotation", "Reset Time", "Stop Move", "Track Front Distance", "Set Lock Angle", "Reset Gyro", "Track Rotation", "Track Lateral Encoders", "NavX Pos Reset", "Track Vision Lat", "Track Vision Rot", "Reset Position"] ("Actions")
      }
      frame "Strafing" {
        n76 = Unbundle By Name(w438) -> ("CMD Drive.CMDMODE"=w437:T4)
        n77 = case shown="\"Strafe Right\"" w437 {
          tunnel: [w440 w441 w443] -> w436
          tunnel: [ENUM_State."Idle" ("State") ENUM_State."Strafing" ("State") ENUM_State."Strafing" ("State")] -> w435
          frame Default {
            w440 = T9[] [enum."No Action"] items=["Drive", "Strafe Left", "Strafe Right", "No Action", "Manuel Keep Rotation", "Reset Time", "Stop Move", "Track Front Distance", "Set Lock Angle", "Reset Gyro", "Track Rotation", "Track Lateral Encoders", "NavX Pos Reset", "Track Vision Lat", "Track Vision Rot", "Reset Position"] ("Actions")
          }
          frame "Strafe Left" {
            w441 = T9[] [enum."Strafe Left"] items=["Drive", "Strafe Left", "Strafe Right", "No Action", "Manuel Keep Rotation", "Reset Time", "Stop Move", "Track Front Distance", "Set Lock Angle", "Reset Gyro", "Track Rotation", "Track Lateral Encoders", "NavX Pos Reset", "Track Vision Lat", "Track Vision Rot", "Reset Position"] ("Actions")
          }
          frame "Strafe Right" {
            w443 = T9[] [enum."Strafe Right"] items=["Drive", "Strafe Left", "Strafe Right", "No Action", "Manuel Keep Rotation", "Reset Time", "Stop Move", "Track Front Distance", "Set Lock Angle", "Reset Gyro", "Track Rotation", "Track Lateral Encoders", "NavX Pos Reset", "Track Vision Lat", "Track Vision Rot", "Reset Position"] ("Actions")
          }
        }
      }
      frame "Halt" {
        (unwired) FALSE
        n78 = Unbundle By Name(w446) -> ("CMD Drive.CMDMODE"=w447:T4)
        n79 = case shown="Default" w447 {
          tunnel: [ENUM_State."Halt" ("State") ENUM_State."Idle" ("State")] -> w445
          tunnel: [w450 w451] -> w448
          frame "Halt" {
            w450 = T9[] [enum."Stop Move"] items=["Drive", "Strafe Left", "Strafe Right", "No Action", "Manuel Keep Rotation", "Reset Time", "Stop Move", "Track Front Distance", "Set Lock Angle", "Reset Gyro", "Track Rotation", "Track Lateral Encoders", "NavX Pos Reset", "Track Vision Lat", "Track Vision Rot", "Reset Position"] ("Actions")
          }
          frame Default {
            w451 = T9[] [enum."Stop Move"] items=["Drive", "Strafe Left", "Strafe Right", "No Action", "Manuel Keep Rotation", "Reset Time", "Stop Move", "Track Front Distance", "Set Lock Angle", "Reset Gyro", "Track Rotation", "Track Lateral Encoders", "NavX Pos Reset", "Track Vision Lat", "Track Vision Rot", "Reset Position"] ("Actions")
          }
        }
      }
    }
    n80 = call "Utility Delay ON.vi"("Delay Time"=w24, "Input"=w25) -> ("Output"=w26:bool)  [unwired: 9 in]
    "Complete" <- w26
    n81 = Unbundle By Name(w42) -> ("CMD Drive.CMDMODE"=w41:T4)
    "CMDMODE" <- w41
    n82 = Bundle By Name(cluster=w42, "Status OUT.Drive Cmd"=w41, "Status OUT.Complete"=w26, "Actions"=w58, "State"=w40) -> (w65:T16)
    n83 = Unbundle By Name(w65) -> ("Actions"=w68:T9[])
    n84 = for {
      tunnel: w68 -> [w76] mode=indexing
      shift-right: [w75] -> w38
      shift-left: w65 -> [w74]
      tunnel: "PID Track Rotation" -> [w73]
      tunnel: "PID Lock Angle Rotation" -> [w72]
      n85 = case shown="\"Manuel Keep Rotation\"" w76 {
        tunnel: w74 -> [w77 w80 w83 w86 w99 w113 w127 w145 w166 w193 w198 w208 w215 w222 w224 w226]
        tunnel: [w77 w79 w82 w85 w100 w114 w130 w151 w169 w194 w197 w207 w214 w221 w224 w226] -> w75
        tunnel: w73 -> [_ _ _ _ w97 _ _ w147 _ w186 _ _ _ _ _ _]
        tunnel: w72 -> [_ _ _ _ _ w103 _ _ _ _ _ _ _ _ _ _]
        frame "No Action" {
        }
        frame "Reset Time" {
          # "Reset timer by taking the current time\nand making it the start time\n\nLater when the current time is \nsubtracted from the start time\nyou will get the elapsed time in \nseconds"
          n86 = Unbundle By Name(w80) -> ("Current Time"=w78:timestamp)
          n87 = Bundle By Name(cluster=w80, "Start Time"=w78) -> (w79:T16)
        }
        frame "Reset Position" {
          n88 = Bundle By Name(cluster=w83, "DriveHWCmd OUT.Reset Postition"=TRUE) -> (w82:T16)
        }
        frame "Stop Move" {
          w84 = 0.0 ("Drive Data.X")
          n89 = Bundle By Name(cluster=w86, "DriveHWCmd OUT.X"=w84, "DriveHWCmd OUT.Y"=w84, "DriveHWCmd OUT.Rotation"=w84) -> (w85:T16)
        }
        frame "Track Rotation" {
          n90 = Unbundle By Name(w99) -> ("CMD Drive.Auto Angle"=w95:dbl, "Gyro Angle"=w96:dbl)
          n91 = call-poly <vilib>:"PID.vi"("output range"=cluster{"output high":dbl, "output low":dbl} {"output high"=0.5, "output low"=-0.5} ("ROITATION range"), "PID gains"=w97, "process variable"=w96, "setpoint"=w95) -> ("output"=w90:dbl)  [unwired: 6 in, 1 out]
          n92 = Sign(1:w90) -> (0:w89:dbl)
          n93 = Multiply(x=0.22, y=w89) -> (x*y=w91:dbl)
          n94 = Add(x=w91, y=w90) -> (x+y=w93:dbl)
          n95 = Bundle By Name(cluster=w99, "DriveHWCmd OUT.HW Mode"=Enum_HW_Cmd_Select."Vbus" ("HWCMD Out.HW Mode"), "PID Target"=w95, "PID Reading"=w96, "PID Output"=w93, "DriveHWCmd OUT.Rotation"=w93, "DriveHWCmd OUT.X"=0.0 ("HWCMD Out.X"), "DriveHWCmd OUT.Y"=0.0 ("HWCMD Out.X"), "PID Select"=Enum_Tab_Select_PID_Mode."Nav Rotation Static") -> (w100:T16)
        }
        frame "Manuel Keep Rotation" {
          n96 = Unbundle By Name(w113) -> ("CMD Drive.Auto Angle"=w106:dbl, "Gyro Angle"=w107:dbl, "CMD Drive.X"=w108:dbl, "CMD Drive.Y"=w109:dbl, "CMD Drive.Speed Divider"=w110:dbl)
          n97 = call-poly <vilib>:"PID.vi"("output range"=cluster{"output high":dbl, "output low":dbl} {"output high"=0.5, "output low"=-0.5} ("ROITATION range"), "PID gains"=w103, "process variable"=w107, "setpoint"=w106) -> ("output"=w104:dbl)  [unwired: 6 in, 1 out]
          n98 = Divide(x=w108, y=w110) -> (x/y=w111:dbl)
          n99 = Divide(x=w109, y=w110) -> (x/y=w112:dbl)
          n100 = Bundle By Name(cluster=w113, "DriveHWCmd OUT.HW Mode"=Enum_HW_Cmd_Select."Vbus" ("HWCMD Out.HW Mode"), "PID Target"=w106, "PID Reading"=w107, "PID Output"=w104, "DriveHWCmd OUT.Rotation"=w104, "DriveHWCmd OUT.X"=w111, "DriveHWCmd OUT.Y"=w112, "PID Select"=Enum_Tab_Select_PID_Mode."Nav Lock Rotation") -> (w114:T16)
        }
        frame "Track Lateral Encoders" {
          w122 = 0.0 ("X Out")
          # "It takes at least .2\nvalue to move lateral\nthis forces a min value of .2\nsame sign as output"
          n101 = Unbundle By Name(w127) -> ("CMD Drive.Target Distance"=w125:dbl, "Lateral Distance"=w126:dbl)
          n102 = call-poly <vilib>:"PID.vi"("output range"=cluster{"output high":dbl, "output low":dbl} {"output high"=0.5, "output low"=-0.5}, "PID gains"="PID Track Lateral", "process variable"=w126, "setpoint"=w125) -> ("output"=w118:dbl)  [unwired: 6 in, 1 out]
          n103 = Sign(1:w118) -> (0:w119:dbl)
          n104 = Multiply(x=0.2, y=w119) -> (x*y=w120:dbl)
          n105 = Add(x=w120, y=w118) -> (x+y=w117:dbl)
          n106 = Bundle By Name(cluster=w127, "DriveHWCmd OUT.HW Mode"=Enum_HW_Cmd_Select."Vbus" ("HWCMD Out.HW Mode"), "DriveHWCmd OUT.Rotation"=w122, "DriveHWCmd OUT.X"=w117, "DriveHWCmd OUT.Y"=w122, "PID Output"=w117, "PID Reading"=w126, "PID Target"=w125, "DriveHWCmd OUT.Reset Postition"=FALSE, "PID Select"=Enum_Tab_Select_PID_Mode."Encoder Lat") -> (w130:T16)
        }
        frame "Track Vision Lat" {
          # "It takes at least .2\nvalue to move lateral\nthis forces a min value of .2\nsame sign as output"
          n107 = Unbundle By Name(w145) -> ("Vision Data.Target Found"=w148:bool, "Vision Data.Vision Distance Center (in)"=w131:dbl)
          n108 = call "Set Max values  from distance location.vi"("Vision Data.Vision Distance Center (in)"=w131) -> ()  [unwired: 10 in, 1 out]
          n109 = Unbundle By Name(w145) -> ("Lock Angle"=w144:dbl, "Gyro Angle"=w143:dbl)
          n110 = case shown="True" w148 {
            tunnel: "PID Track Vision Lat" -> [_ w157]
            tunnel: [0.0 ("output") w156] -> w132
            tunnel: w131 -> [_ w154]
            tunnel: [_ w155] -> w141
            tunnel: [_ w154] -> w140
            tunnel: cluster{"output high":dbl, "output low":dbl} {"output high"=0.5, "output low"=-0.5} ("output range") -> [_ w153]
            frame False {
            }
            frame True {
              w155 = 0.0 ("setpoint")
              n111 = call-poly <vilib>:"PID.vi"("output range"=w153, "PID gains"=w157, "process variable"=w154, "setpoint"=w155) -> ("output"=w156:dbl)  [unwired: 6 in, 1 out]
            }
          }
          n112 = call-poly <vilib>:"PID.vi"("output range"=cluster{"output high":dbl, "output low":dbl} {"output high"=1.0, "output low"=-1.0}, "PID gains"=w147, "process variable"=w143, "setpoint"=w144) -> ("output"=w142:dbl)  [unwired: 6 in, 1 out]
          n113 = Sign(1:w132) -> (0:w134:dbl)
          n114 = Multiply(x="lateral f", y=w134) -> (x*y=w135:dbl)
          n115 = Add(x=w135, y=w132) -> (x+y=w133:dbl)
          n116 = Bundle By Name(cluster=w145, "DriveHWCmd OUT.HW Mode"=Enum_HW_Cmd_Select."Vbus" ("HWCMD Out.HW Mode"), "PID Target"=w141, "PID Reading"=w140, "PID Output"=w133, "DriveHWCmd OUT.Rotation"=w142, "DriveHWCmd OUT.X"=w133, "DriveHWCmd OUT.Y"=0.0 ("X Out"), "PID Select"=Enum_Tab_Select_PID_Mode."Vision Lateral") -> (w151:T16)
        }
        frame "Track Vision Rot" {
          w159 = 0.0 ("X Out")
          # "#Vision_LOCATION_PID  Location To PID setting HERE"
          n117 = Unbundle By Name(w166) -> ("Vision Data.Target Found"=w167:bool, "Vision Data.Angle Distance Center (in)"=w161:dbl)
          n118 = disable-structure shown="Disabled" {
            disable-tunnel: w161 -> [w170 _]
            frame Disabled {
              n119 = call "Set Max values  from distance location.vi"("Vision Data.Vision Distance Center (in)"=w170) -> ()  [unwired: 10 in, 1 out]
            }
            frame Enabled {
            }
          }
          n120 = case shown="True" w167 {
            tunnel: "PID Track Vision Rot" -> [_ w180]
            tunnel: [0.0 ("output") w172] -> w160
            tunnel: w161 -> [_ w178]
            tunnel: [_ "Vision Track target"] -> w165
            tunnel: [_ w178] -> w164
            tunnel: cluster{"output high":dbl, "output low":dbl} {"output high"=0.5, "output low"=-0.5} ("output range") -> [_ w177]
            frame False {
            }
            frame True {
              n121 = call-poly <vilib>:"PID.vi"("output range"=w177, "PID gains"=w180, "process variable"=w178, "setpoint"="Vision Track target") -> ("output"=w174:dbl)  [unwired: 6 in, 1 out]
              n122 = Sign(1:w174) -> (0:w176:dbl)
              n123 = Multiply(x=0.25, y=w176) -> (x*y=w173:dbl)
              n124 = Add(x=w174, y=w173) -> (x+y=w172:dbl)
            }
          }
          n125 = Bundle By Name(cluster=w166, "DriveHWCmd OUT.HW Mode"=Enum_HW_Cmd_Select."Vbus" ("HWCMD Out.HW Mode"), "PID Target"=w165, "PID Reading"=w164, "PID Output"=w159, "DriveHWCmd OUT.Rotation"=w160, "DriveHWCmd OUT.X"=w159, "DriveHWCmd OUT.Y"=w159, "PID Select"=Enum_Tab_Select_PID_Mode."Vision Rotation") -> (w169:T16)
        }
        frame "Track Front Distance" {
          n126 = Unbundle By Name(w193) -> ("Lock Angle"=w191:dbl, "Gyro Angle"=w192:dbl, "CMD Drive.Target Distance"=w183:dbl, "Sonar Distance"=w181:dbl)
          n127 = call-poly <vilib>:"PID.vi"("output range"=cluster{"output high":dbl, "output low":dbl} {"output high"=1.0, "output low"=-1.0}, "PID gains"=w186, "process variable"=w192, "setpoint"=w191) -> ("output"=w190:dbl)  [unwired: 6 in, 1 out]
          n128 = call-poly <vilib>:"PID.vi"("output range"=cluster{"output high":dbl, "output low":dbl} {"output high"=0.5, "output low"=-0.5}, "PID gains"="PID Track Front", "process variable"=w181, "setpoint"=w183) -> ("output"=w185:dbl)  [unwired: 6 in, 1 out]
          n129 = Bundle By Name(cluster=w193, "DriveHWCmd OUT.HW Mode"=Enum_HW_Cmd_Select."Vbus" ("HWCMD Out.HW Mode"), "DriveHWCmd OUT.Rotation"=w190, "DriveHWCmd OUT.X"=0.0 ("X Out"), "DriveHWCmd OUT.Y"=w185, "PID Output"=w185, "PID Target"=w183, "PID Reading"=w181, "PID Select"=Enum_Tab_Select_PID_Mode."Sonar Front") -> (w194:T16)
        }
        frame "Set Lock Angle" {
          n130 = Unbundle By Name(w198) -> ("Gyro Angle"=w196:dbl)
          n131 = Bundle By Name(cluster=w198, "Lock Angle"=w196) -> (w197:T16)
        }
        frame "Drive" {
          n132 = Unbundle By Name(w208) -> ("CMD Drive.X"=w200:dbl, "CMD Drive.Y"=w202:dbl, "CMD Drive.Rotation"=w203:dbl, "CMD Drive.Speed Divider"=w201:dbl)
          n133 = Divide(x=w200, y=w201) -> (x/y=w206:dbl)
          n134 = Divide(x=w202, y=w201) -> (x/y=w205:dbl)
          n135 = Divide(x=w203, y=w201) -> (x/y=w204:dbl)
          n136 = Bundle By Name(cluster=w208, "DriveHWCmd OUT.HW Mode"=Enum_HW_Cmd_Select."Vbus" ("HWCMD Out.HW Mode"), "DriveHWCmd OUT.X"=w206, "DriveHWCmd OUT.Y"=w205, "DriveHWCmd OUT.Rotation"=w204) -> (w207:T16)
        }
        frame "Strafe Left" {
          n137 = Bundle By Name(cluster=w215, "DriveHWCmd OUT.HW Mode"=Enum_HW_Cmd_Select."Vbus" ("HWCMD Out.HW Mode"), "DriveHWCmd OUT.X"=-1.0, "DriveHWCmd OUT.Y"=0.0, "DriveHWCmd OUT.Rotation"=0.0, "DriveHWCmd OUT.Angle"=0.0) -> (w214:T16)
        }
        frame "Strafe Right" {
          n138 = Bundle By Name(cluster=w222, "DriveHWCmd OUT.HW Mode"=Enum_HW_Cmd_Select."Vbus" ("HWCMD Out.HW Mode"), "DriveHWCmd OUT.X"=1.0, "DriveHWCmd OUT.Y"=0.0, "DriveHWCmd OUT.Rotation"=0.0, "DriveHWCmd OUT.Angle"=0.0) -> (w221:T16)
        }
        frame "Reset Gyro" {
          n139 = call <vilib>:"Zero Yaw.vi"("Device Number"=FRIC_navX_DeviceNumbersTypeDef."Dev0") -> ()  [unwired: 11 in]
        }
        frame "NavX Pos Reset" {
          n140 = call <vilib>:"Zero Displacement.vi"("Device Number"=FRIC_navX_DeviceNumbersTypeDef."Dev0") -> ()  [unwired: 11 in]
        }
      }
      "Action" <- w76
    }
    n141 = Unbundle By Name(w38) -> ("DriveHWCmd OUT"=w56:T5, "Status OUT"=w43:T12, "PID Select"=w28:T7)
    "HW Cmd Out" <- w56
    n142 = Unbundle By Name(w38) -> ("PID Target"=w36:dbl, "PID Reading"=w35:dbl, "PID Output"=w37:dbl)
    "PID Target" <- w36
    "PID Reading" <- w35
    "PID Output" <- w37
    n143 = global write "Global_SM Out Data.vi" "Drive_SM_HWCmd"(w56) -> ()
    n144 = Bundle("PID Target"=w36, "PID Reading"=w35) -> (w34:cluster{"PID Target":dbl, "PID Reading":dbl})  [unwired: 1 in]
    n145 = global write "Global_SM Out Data.vi" "Drive_SM_Status"(w43) -> ()
    n146 = local write "PID Select"(w28) -> ()
    n147 = Bundle By Name(cluster=w38, "previous State"=w45) -> (w48:T16)
    n148 = flat-sequence {
      tunnel: w37 -> [w71]
      tunnel: w34 -> [w70]
      tunnel: [w69] -> w32
      frame #0 {
        n149 = Get Date/Time In Seconds() -> (seconds since 1Jan1904=w69:timestamp)
        "Process Chart" <- w70
        "Output" <- w71
      }
    }
    n150 = feedback-in #1(w32) -> ()
    n151 = feedback #1() -> (w33:timestamp)  [unwired: 1 in]
    n152 = Subtract(x=w32, y=w33) -> (x-y=→"Cycle Time":dbl)
  }
  n153 = call "Utility Delay ON.vi"() -> ()  [unwired: 11 in, 1 out]
